vi "Ack Completion With Error.vi"(8 "error in (no error)":errorcluster, 10 "Completion Ack Data":T1, 11 "Async Methods Actor Example in":refnum<class "Async Methods Actor Example.lvclass">) -> (0 "error out":errorcluster, 3 "Async Methods Actor Example out":refnum<class "Async Methods Actor Example.lvclass">)   [LabVIEW 2023, in "Async Methods Actor Example.lvlib" / "Async Methods Actor Example.lvclass"]
uses:
  Async Methods Actor Example.lvclass
  Async Methods Actor/Async Methods Actor Messages/Completion Notification Msg/Completion Notification Data.ctl
  Async Methods Actor/Async Methods Actor Messages/Async Message/Async Message.lvclass
  Async Methods Actor Example.lvclass/Async Methods Actor Example.ctl
  Async Methods Actor/Async Methods Actor Messages/Completion Notification Msg/Completion Notification Msg.lvclass
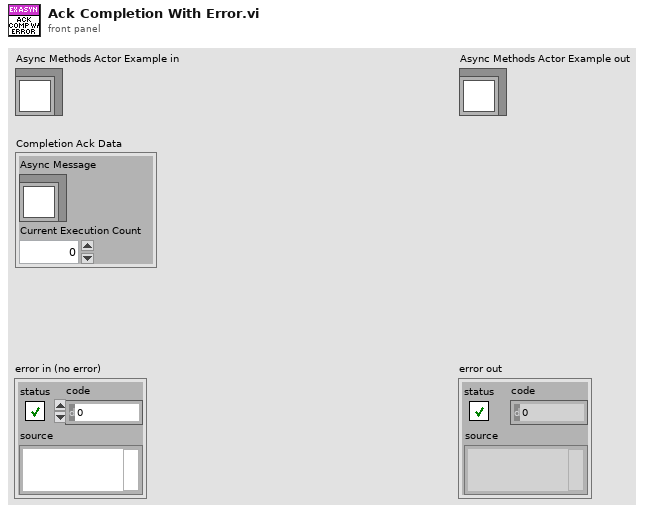
[diagram p1: front panel]
types:
  T1 = typedef "Async Methods Actor.lvlib/Completion Notification Msg.lvclass/Completion Notification Data.ctl" = cluster{"Async Message":refnum<class "Async Message.lvclass">, "Current Execution Count":u32}
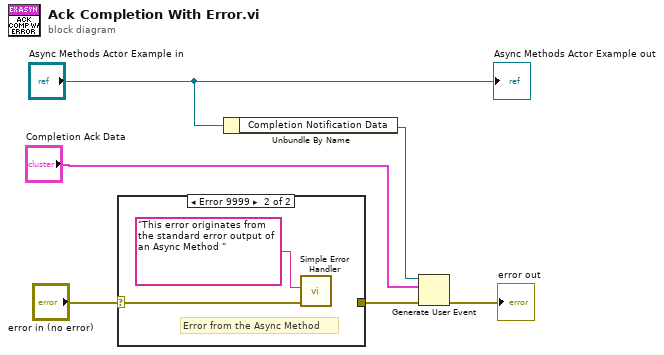
[diagram p0: block diagram]
diagram:
  n1 = case shown="Error 9999" "error in (no error)" {
    selector: "error in (no error)" -> [w7 w9]
    tunnel: [w7 _] -> w1
    frame No Error {
    }
    frame Error {
      # "Error from the Async Method"
      n2 = call <vilib>:"Simple Error Handler.vi"("error source (\" \")"="This error originates from the standard error output of an Async Method " ("error source (\" \")"), "error in (no error)"=w9) -> ()  [unwired: 3 in, 5 out]
    }
  }
  n3 = Unbundle By Name("Async Methods Actor Example in") -> ("Completion Notification Data"=w4:refnum<user-event>)
  n4 = Generate User Event(user event=w4, event data cluster="Completion Ack Data", error in=w1) -> (error out=→"error out":errorcluster)  [unwired: 1 in, 1 out]
  "Async Methods Actor Example out" <- "Async Methods Actor Example in"
